vi "LinxOpen.vi"(8 "Error In":errorcluster) -> (0 "Error Out":errorcluster, 3 "LINX Resource":T1)   [LabVIEW 2020, in "LMH-LINX.lvlib" / "Local IO.lvlib"]
uses:
  Local IO.lvlib
  Type Defs/LINX Ref.ctl
  Type Defs/Platform.ctl
  Type Defs/Interface.ctl
  Device/Type Defs/LINX Device Config.ctl
  Device/Type Defs/TCP Config.ctl
  Device/Type Defs/Channels.ctl
  Type Defs/Error Type.ctl
  LMH-LINX.lvlib
  <vilib>/MakerHub/LINX/Private/Type Defs/Channel FGV States.ctl
  Device/Device.lvlib
  <vilib>/MakerHub/LINX/Resources/liblinxdevice.dll
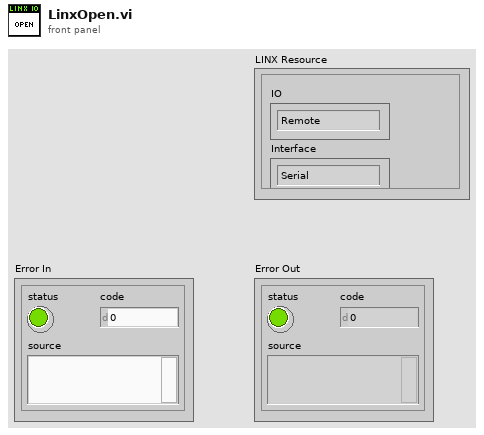
[diagram p1: front panel]
types:
  T1 = typedef "LMH-LINX.lvlib/LINX Ref.ctl" = cluster{"IO":T2, "Interface":T3, "LINX Device Config":T4}
  T2 = typedef "LMH-LINX.lvlib/Platform.ctl" = enum16{"Remote", "Local"}
  T3 = typedef "LMH-LINX.lvlib/Interface.ctl" = enum16{"Serial", "TCP"}
  T4 = typedef "LMH-LINX.lvlib/Device.lvlib/LINX Device Config.ctl" = cluster{"Interface":T3, "COM Port":refnum<visa-resource-name>, "TCP Configuration":T5, "Device Family":u8, "Device ID":u8, "Device Name":string, "TCP Ref":refnum<k5>, "Channels":T6}
  T5 = typedef "LMH-LINX.lvlib/Device.lvlib/TCP Config.ctl" = cluster{"IP Address":string, "Port":u16}
  T6 = typedef "LMH-LINX.lvlib/Channels.ctl" = cluster{"DI":u8[], "DO":u8[], "AI":u8[], "AO":u8[], "PWM":u8[], "QE":u8[], "UART":u8[], "I2C 2":u8[], "SPI":u8[], "CAN":u8[], "Servo":u8[], "AI Ref (V)":dbl, "AI Resolution (Bits)":u8, "AO Ref (V)":dbl, "AO Resolution (Bits)":u8}
  T7 = typedef "LMH-LINX.lvlib/Error Type.ctl" = enum16{"Unknown", "Timeout", "Corrupt Return Packet", "Unable To Connect", "Command Not Supported", "Channel DNE", "Invalid COM Config", "Firmware Version Mismatch", "myRIO Support", "CMD Specific Error", "Local IO Not Supported"}
  T8 = typedef "LMH-LINX.lvlib/Channel FGV States.ctl" = enum16{"Initialize", "Get", "Set"}
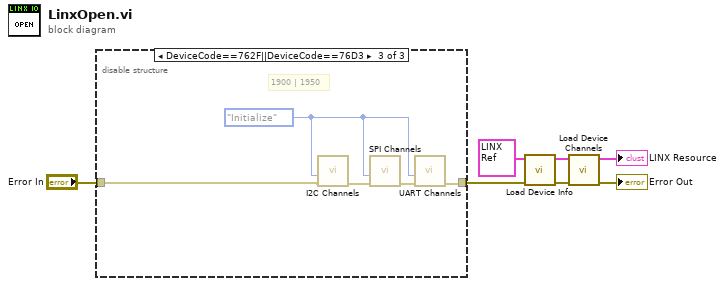
[diagram p0: block diagram]
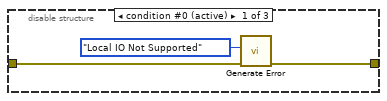
[diagram p2: hidden frame]
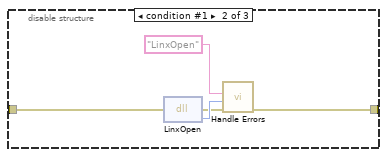
[diagram p3: hidden frame]
diagram:
  n1 = disable-structure shown="DeviceCode==762F||DeviceCode==76D3" {
    disable-tunnel: [w8 w12 w17] -> w5
    disable-tunnel: "Error In" -> [w9 w11 w16]
    frame condition #0 (active) {
      n2 = call "Generate Error.vi"("Error In"=w9, "Error Type"=Error_Type."Local IO Not Supported") -> ("Error Out"=w8:errorcluster)  [unwired: 8 in, 1 out]
    }
    frame condition #1 {
      n3 = dll-call lib="E:/lv2019/dist/vi.lib/MakerHub/LINX/Resources/liblinxdevice.*" fn="LinxOpen"(error in=w11) -> (error out=w13:errorcluster, "LinxStatus"=w14:i32)  [unwired: 2 in, 1 out]
      n4 = call <vilib>:"Handle Errors.vi"("Error In"=w13, "LinxStatus"=w14, "Function Name"="LinxOpen") -> ("Error Out"=w12:errorcluster)  [unwired: 7 in, 1 out]
    }
    frame condition #2 {
      w18 = Channel_FGV_States."Initialize" ("Channel State")
      # "1900 | 1950"
      n5 = call <vilib>:"I2C Channels.vi"("Error In"=w16, "Channel State"=w18) -> ("Error Out"=w20:errorcluster)  [unwired: 8 in, 1 out]
      n6 = call <vilib>:"SPI Channels.vi"("Error In"=w20, "Channel State"=w18) -> ("Error Out"=w19:errorcluster)  [unwired: 8 in, 1 out]
      n7 = call <vilib>:"UART Channels.vi"("Error In"=w19, "Channel State"=w18) -> ("Error Out"=w17:errorcluster)  [unwired: 8 in, 1 out]
    }
  }
  n8 = call "Load Device Info.vi"("Error In"=w5, "LINX Resource"=T1 {"IO"=enum."Remote", "Interface"=enum."Serial", "LINX Device Config"={"Interface"=enum."Serial", "COM Port"="", "TCP Configuration"={"IP Address"="", "Port"=0}, "Device Family"=0, "Device ID"=0, "Device Name"="", "TCP Ref"=refnum, "Channels"={"DI"=[], "DO"=[], "AI"=[], "AO"=[], "PWM"=[], "QE"=[], "UART"=[], "I2C 2"=[], "SPI"=[], "CAN"=[], "Servo"=[], "AI Ref (V)"=0.0, "AI Resolution (Bits)"=0, "AO Ref (V)"=0.0, "AO Resolution (Bits)"=0}}}) -> ("Error Out"=w4:errorcluster, "LINX Resource"=w3:T1)  [unwired: 8 in]
  n9 = call "Load Device Channels.vi"("Error In"=w4, "LINX Resource"=w3) -> ("Error Out"=→"Error Out":errorcluster, "LINX Resource"=→"LINX Resource":T1)  [unwired: 8 in]
